vi "Release Lock.vi"(8 "error in (no error)":errorcluster, 9 "timeout (0 ms)":i32 format="%d ms", 10 "new lock status (T)":bool=TRUE, 11 "Protected Pointer in":refnum<class "Protected Pointer.lvclass">) -> (0 "error out":errorcluster, 1 "timed out?":bool, 3 "Protected Pointer out":refnum<class "Protected Pointer.lvclass">)   [LabVIEW 2017, in "Memory Manager.lvlib" / "Protected Pointer.lvclass"]
uses:
  Protected Pointer.lvclass
  Invalid Lock.vi
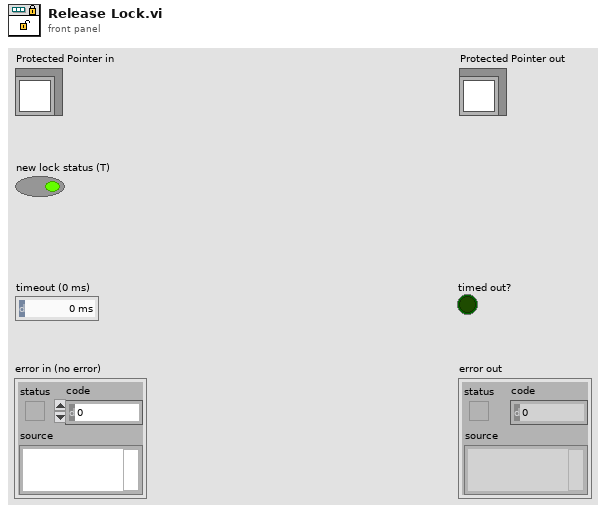
[diagram p1: front panel]
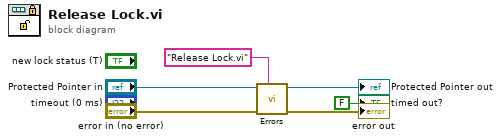
[diagram p0: block diagram]
diagram:
  n1 = call-poly "Errors.vi"("source vi name"="Release Lock.vi", "error in (no error)"="error in (no error)", "Lockable Pointer in"="Protected Pointer in") -> ("error out"=→"error out":errorcluster, "Lockable Pointer out"=→"Protected Pointer out":refnum<class "Protected Pointer.lvclass">)  [unwired: 7 in]
  "timed out?" <- FALSE ("timed out?")
